vi "OptionSelect2.vi"() -> ()   [LabVIEW 2015]
panel:
  in  "stop":bool
  out "Ring 2":u16
  out "Enum 2":enum16{"$5", "$10", "$20", "$100"}(ring)
  in  "Enum":enum16{"$5", "$10", "$20", "$100"}(ring)
  in  "Ring":u16(ring) items=["$5", "$10", "$20", "$100"]
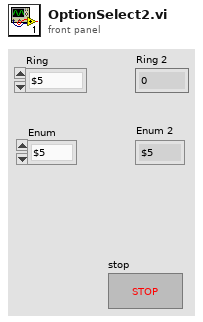
[diagram p1: front panel]
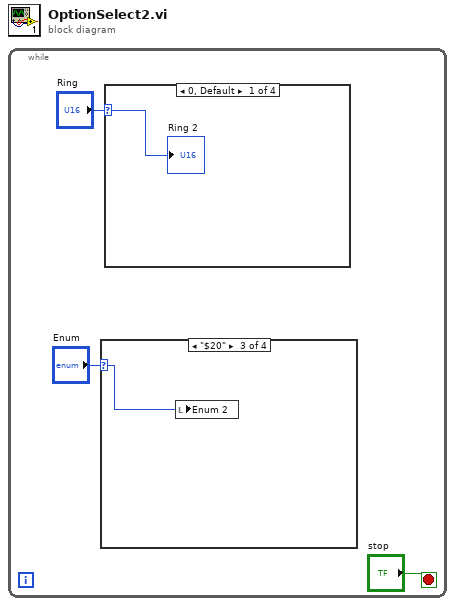
[diagram p0: block diagram]
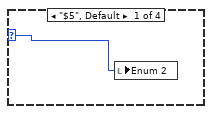
[diagram p2: hidden frame]
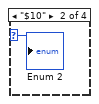
[diagram p3: hidden frame]
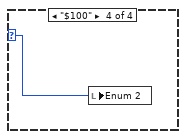
[diagram p4: hidden frame]
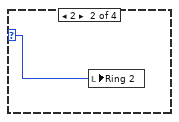
[diagram p5: hidden frame]
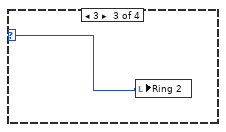
[diagram p6: hidden frame]
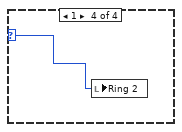
[diagram p7: hidden frame]
diagram:
  n1 = while {
    stop <- "stop" stop-if-true
    n2 = case shown="\"$20\"" "Enum" {
      selector: "Enum" -> [w4 w5 w6 w7]
      frame "$5", Default {
        n3 = local write "Enum 2"(w4) -> ()
      }
      frame "$10" {
        "Enum 2" <- w5
      }
      frame "$20" {
        n4 = local write "Enum 2"(w6) -> ()
      }
      frame "$100" {
        n5 = local write "Enum 2"(w7) -> ()
      }
    }
    n6 = case shown="0, Default" "Ring" {
      selector: "Ring" -> [w8 w9 w10 w11]
      frame 0, Default {
        "Ring 2" <- w8
      }
      frame 2 {
        n7 = local write "Ring 2"(w9) -> ()
      }
      frame 3 {
        n8 = local write "Ring 2"(w10) -> ()
      }
      frame 1 {
        n9 = local write "Ring 2"(w11) -> ()
      }
    }
  }
